vi "LINX - Switch to WiFi.vi"() -> ()   [LabVIEW 2019]
uses:
  <vilib>/MakerHub/LINX/Private/Type Defs/Interface.ctl
  <vilib>/MakerHub/LINX/Private/Device/Type Defs/Wifi Config.ctl
  <vilib>/MakerHub/LINX/Private/Type Defs/WIFI Security Type.ctl
  vi.lib/LINXx/Private/WiFi101 Status.ctl
  <vilib>/MakerHub/LINX/Private/Device/Type Defs/TCP Config.ctl
  vi.lib/LINXx/Public/Reset Target.ctl
  <vilib>/MakerHub/LINX/Public/Peripherals/Digital/Digital Write 1 Chan.vi
  <vilib>/MakerHub/LINX/Public/Peripherals/Digital/Digital Write N Chans.vi
  <vilib>/MakerHub/LINX/Private/Local IO/LinxDigitalWrite.vi
  <vilib>/MakerHub/LINX/Public/Utilities/Check Channel.vi
  <vilib>/MakerHub/LINX/Public/Utilities/Open Serial.vi
  <vilib>/MakerHub/LINX/Private/Utilties/Generate Error.vi
  <vilib>/MakerHub/LINX/LMH-LINX.lvlib
  <vilib>/MakerHub/LINX/Private/Device/Device.lvlib
  vi.lib/LINXx/LINXx.lvlib
panel:
  in  "Reset Board":bool
  in  "Reset WiFI":bool
  out "WiFi Status":T1 items=["No module"=255, "Idle"=0, "No SSID"=1, "Scan completed"=2, "Connected"=3, "Connection failed"=4, "Connection lost"=5, "Disconnected"=6, "AP listening"=7, "AP connected"=8, "AP failed"=9, "Provisioning"=10, "Provisioning failed"=11]
  out "Loop Rate (Hz)":u32
  in  "stop":bool
  in  "New Wifi Config":T2={"SSID"="", "IP Address"="", "Port"=0, "WIFI Security Type"=enum."WPA2 Password", "Password"=""}
  out "Saved Wifi Configuration":T2={"SSID"="", "IP Address"="", "Port"=0, "WIFI Security Type"=enum."WPA2 Password", "Password"=""}
  out "Current connection":T4
  in  "Switch to WiFi connection":bool
  in  "Set WiFi info":bool
  in  "Get WiFi info":bool
  in  "Serial Port":refnum<visa-resource-name>="N/A"
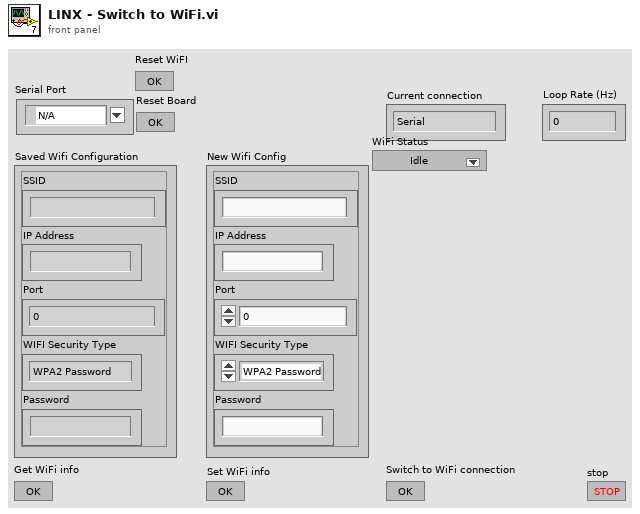
[diagram p1: front panel]
types:
  T1 = typedef "LINXx.lvlib/WiFi101 Status.ctl" = u8
  T2 = typedef "LMH-LINX.lvlib/Device.lvlib/Wifi Config.ctl" = cluster{"SSID":string, "IP Address":string, "Port":u16, "WIFI Security Type":T3, "Password":string}
  T3 = typedef "LMH-LINX.lvlib/WIFI Security Type.ctl" = enum8{"None", "WPA2 Password", "WPA2 Key", "WEP40", "WEP104"}
  T4 = typedef "LMH-LINX.lvlib/Interface.ctl" = enum16{"Serial", "TCP"}
  T5 = typedef "LMH-LINX.lvlib/LINX Ref.ctl" = cluster{"IO":T6, "Interface":T4, "LINX Device Config":T7}
  T6 = typedef "LMH-LINX.lvlib/Platform.ctl" = enum16{"Remote", "Local"}
  T7 = typedef "LMH-LINX.lvlib/Device.lvlib/LINX Device Config.ctl" = cluster{"Interface":T4, "COM Port":refnum<visa-resource-name>, "TCP Configuration":T8, "Device Family":u8, "Device ID":u8, "Device Name":string, "TCP Ref":refnum<k5>, "Channels":T9}
  T8 = typedef "LMH-LINX.lvlib/Device.lvlib/TCP Config.ctl" = cluster{"IP Address":string, "Port":u16}
  T9 = typedef "LMH-LINX.lvlib/Channels.ctl" = cluster{"DI":u8[], "DO":u8[], "AI":u8[], "AO":u8[], "PWM":u8[], "QE":u8[], "UART":u8[], "I2C 2":u8[], "SPI":u8[], "CAN":u8[], "Servo":u8[], "AI Ref (V)":dbl, "AI Resolution (Bits)":u8, "AO Ref (V)":dbl, "AO Resolution (Bits)":u8}
  T10 = typedef "LINXx.lvlib/Reset Target.ctl" = enum16{"None", "Serial", "TCP", "Board"}
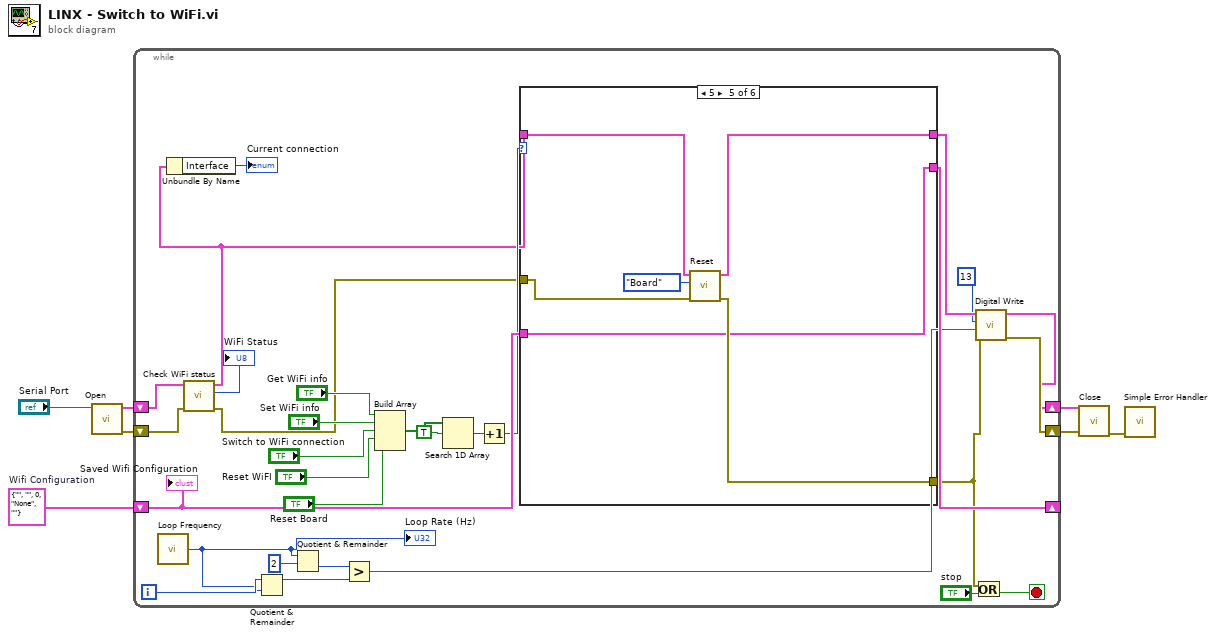
[diagram p0: block diagram]
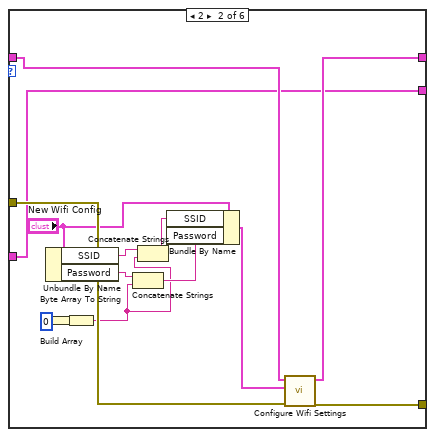
[diagram p3: hidden frame]
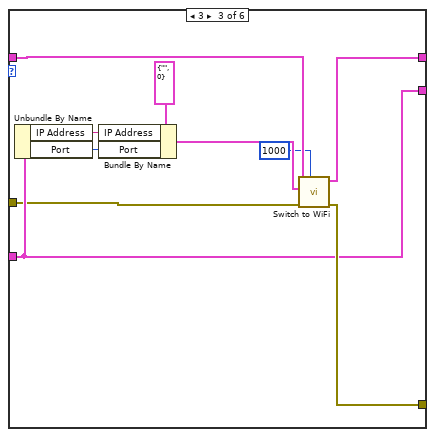
[diagram p4: hidden frame]
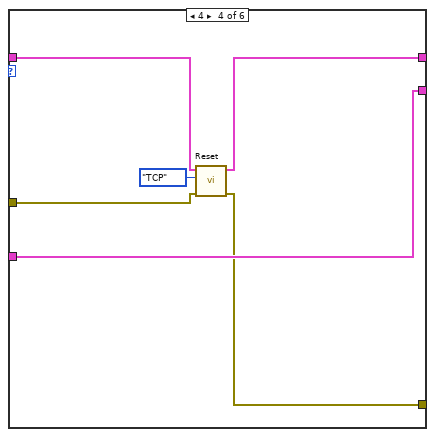
[diagram p5: hidden frame]
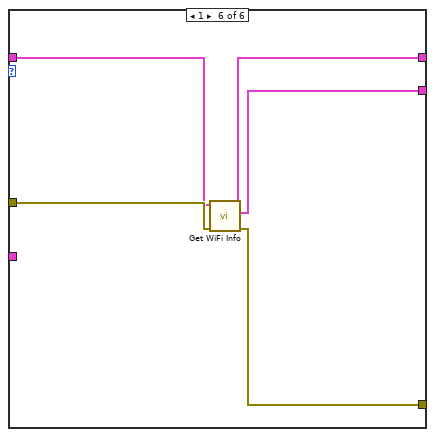
[diagram p6: hidden frame]
diagram:
  w4 = T2 {"SSID"="", "IP Address"="", "Port"=0, "WIFI Security Type"=enum."None", "Password"=""}  # Wifi Configuration
  n1 = call-poly <vilib>:"Open.vi"("Serial Port"="Serial Port") -> ("Error Out"=w5:errorcluster, "LINX Resource"=w6:T5)  [unwired: 8 in, 1 out]
  n2 = while {
    shift-right: [w23] -> w2
    shift-left: w6 -> [w17]
    shift-right: [w24] -> w3
    shift-left: w5 -> [w14]
    shift-right: [w35] -> _
    shift-left: w4 -> [w36]
    i -> [w20]
    stop <- w26 stop-if-true
    n3 = call <vilib>:"Loop Frequency.vi"() -> ("Loop Rate (Hz)"=w12:u32)
    "Loop Rate (Hz)" <- w12
    n4 = call "Check WiFi status.vi"("Error In"=w14, "LINX Resource"=w17) -> ("Error Out"=w13:errorcluster, "WiFi status"=→"WiFi Status":u8, "LINX Resource out"=w16:T5)  [unwired: 7 in]
    n5 = Unbundle By Name(w16) -> ("Interface"=→"Current connection":T4)
    n6 = Quotient & Remainder(x=w20, y=w12) -> (x-y*floor(x/y)=w19:u32)  [unwired: 1 out]
    n7 = Quotient & Remainder(x=w12, y=u32 2) -> (floor(x/y)=w10:u32)  [unwired: 1 out]
    n8 = Greater?(x=w10, y=w19) -> (0:w18:bool)
    n9 = Build Array("Get WiFi info", "Set WiFi info", "Switch to WiFi connection", "Reset WiFI", "Reset Board") -> (w31:bool[])
    n10 = Search 1D Array(1D array=w31, element=TRUE) -> (index of element=w29:i32)  [unwired: 1 in]
    n11 = Increment(x=w29) -> (x+1=w28:i32)
    n12 = case shown="5" w28 {
      tunnel: w36 -> [w40 w50 w60 w70 w72 _]
      tunnel: [w40 w50 w60 w70 w72 w77] -> w35
      tunnel: w13 -> [w39 w54 w57 w69 w76 w81]
      tunnel: [w39 w53 w63 w68 w73 w80] -> w22
      tunnel: w16 -> [w38 w52 w56 w67 w75 w79]
      tunnel: [w38 w51 w64 w65 w74 w78] -> w25
      frame 0, Default {
      }
      frame 2 {
        n13 = Unbundle By Name("New Wifi Config") -> ("SSID"=w42:string, "Password"=w47:string)
        n14 = Build Array(u8 0) -> (w45:u8[])
        n15 = Byte Array To String(unsigned byte array=w45) -> (string=w41:string)
        n16 = Concatenate Strings(w47, w41) -> (w43:string)
        n17 = Concatenate Strings(w42, w41) -> (w44:string)
        n18 = Bundle By Name(cluster="New Wifi Config", "SSID"=w44, "Password"=w43) -> (w49:T2)
        n19 = call <vilib>:"Configure Wifi Settings.vi"("Error In"=w54, "Wifi Configuration"=w49, "LINX Resource"=w52) -> ("Error Out"=w53:errorcluster, "LINX Resource"=w51:T5)  [unwired: 7 in]
      }
      frame 3 {
        n20 = Unbundle By Name(w60) -> ("IP Address"=w59:string, "Port"=w58:u16)
        n21 = Bundle By Name(cluster=T8 {"IP Address"="", "Port"=0} ("TCP Configuration"), "IP Address"=w59, "Port"=w58) -> (w61:T8)
        n22 = call "Switch to WiFi.vi"("Retry wait time [ms]"=u32 1000, "Error In"=w57, "TCP Configuration"=w61, "LINX Resource"=w56) -> ("Error Out"=w63:errorcluster, "LINX Resource out"=w64:T5)  [unwired: 6 in]
      }
      frame 4 {
        n23 = call "Reset.vi"("Error In"=w69, "Reset Target"=Reset_Target."TCP", "LINX Resource"=w67) -> ("Error Out"=w68:errorcluster, "LINX Resource out"=w65:T5)  [unwired: 7 in]
      }
      frame 5 {
        n24 = call "Reset.vi"("Error In"=w76, "Reset Target"=Reset_Target."Board", "LINX Resource"=w75) -> ("Error Out"=w73:errorcluster, "LINX Resource out"=w74:T5)  [unwired: 7 in]
      }
      frame 1 {
        n25 = call "Get WiFi Info.vi"("Error In"=w81, "LINX Resource"=w79) -> ("Error Out"=w80:errorcluster, "WiFi Info"=w77:T2, "LINX Resource Out"=w78:T5)  [unwired: 6 in, 1 out]
      }
    }
    n26 = Or(x=w22, y="stop") -> (x .or. y?=w26:bool)
    n27 = call-poly <vilib>:"Digital Write.vi"("Error In"=w22, "Output Value"=w18, "DO Channel"=u8 13, "LINX Resource"=w25) -> ("Error Out"=w24:errorcluster, "LINX Resource"=w23:T5)  [unwired: 6 in]
    "Saved Wifi Configuration" <- w36
  }
  n28 = call <vilib>:"Close.vi"("Error In"=w3, "LINX Resource"=w2) -> ("Error Out"=w1:errorcluster)  [unwired: 9 in]
  n29 = call <vilib>:"Simple Error Handler.vi"("error in (no error)"=w1) -> ()  [unwired: 4 in, 5 out]
